vi "Tool Q LEIN High G  Start.vi"(0 "Controller ID":u8=42, 5 "G trigger limit(5 G)":dbl=5.0, 9 "Numb pre samples(250)":u16=250, 11 "error in (no error)":errorcluster) -> (4 "LEIN custom reply Q":T1, 15 "error out":errorcluster)   [LabVIEW 2011]
uses:
  LEINmaster/Defenitions/LEIN custom reply Q.ctl
  LEINmaster/Defenitions/LEIN Reply Holder.ctl
  LEINmaster/Defenitions/LEIN CMD Cluster.ctl
  LEINmaster/Defenitions/LEIN CMD List.ctl
  LEINmaster/Defenitions/LEIN Structure variations.ctl
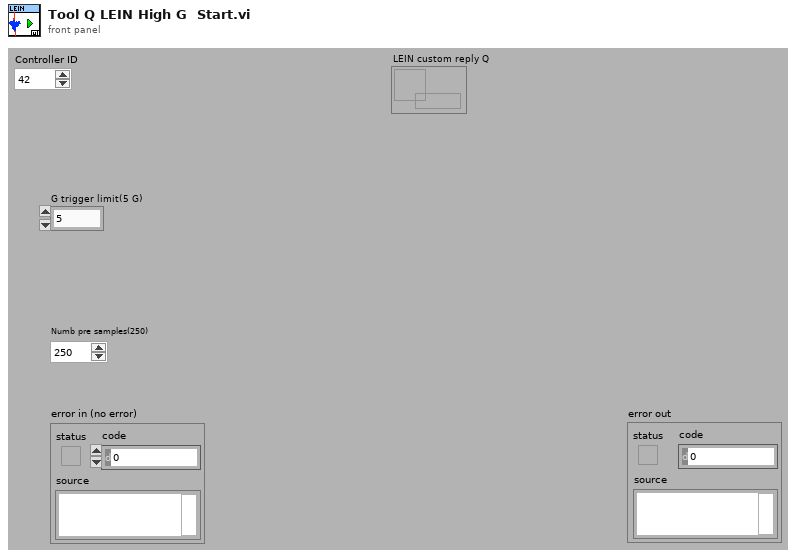
[diagram p1: front panel]
types:
  T1 = typedef "LEIN custom reply Q.ctl" = refnum<queue>
  T2 = typedef "LEIN Structure variations.ctl" = enum16{"LEIN08", "LEIN31", "LEIN63"}
  T3 = enum16{"big-endian, network order", "native, host order", "little-endian"}
  T4 = typedef "LEIN CMD Cluster.ctl" = cluster{"SID":u8, "ANF":bool, "CMD":T5, "DATA":u8[]}
  T5 = typedef "LEIN CMD List.ctl" = enum8{"ACTI", "TASK", "RES0", "STAT", "RES1", "RES2", "RES3", "USER"}
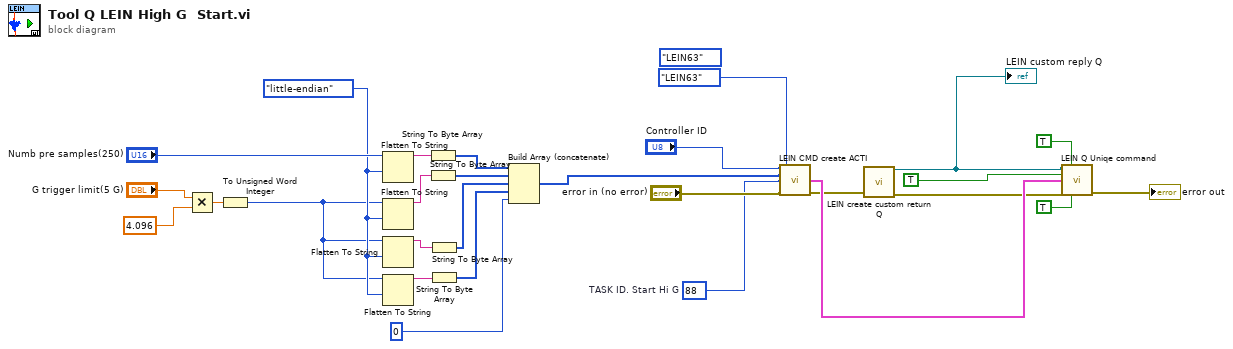
[diagram p0: block diagram]
diagram:
  (unwired) LEIN_Structure_variations."LEIN63" ("LEIN Variation")
  w7 = u8 88  # TASK ID. Start Hi G
  w14 = T3."little-endian" ("byte order (0:big-endian, network order)")
  n1 = Multiply(x="G trigger limit(5 G)", y=4.096 ("x")) -> (x*y=w27:dbl)
  n2 = To Unsigned Word Integer(number=w27) -> (unsigned 16bit integer=w13:u16)
  n3 = Flatten To String(anything="Numb pre samples(250)", byte order (0:big-endian, network order)=w14) -> (data string=w25:string)  [unwired: 2 in, 2 out]
  n4 = Flatten To String(anything=w13, byte order (0:big-endian, network order)=w14) -> (data string=w23:string)  [unwired: 2 in, 2 out]
  n5 = Flatten To String(anything=w13, byte order (0:big-endian, network order)=w14) -> (data string=w17:string)  [unwired: 2 in, 2 out]
  n6 = Flatten To String(anything=w13, byte order (0:big-endian, network order)=w14) -> (data string=w16:string)  [unwired: 2 in, 2 out]
  n7 = String To Byte Array(string=w25) -> (unsigned byte array=w24:u8[])
  n8 = String To Byte Array(string=w23) -> (unsigned byte array=w22:u8[])
  n9 = String To Byte Array(string=w17) -> (unsigned byte array=w18:u8[])
  n10 = String To Byte Array(string=w16) -> (unsigned byte array=w15:u8[])
  n11 = Build Array (concatenate)(w24, w22, w18, w15, u8 0) -> (w8:u8[])
  n12 = call "LEIN CMD create ACTI.vi"("SID"="Controller ID", "LEIN Variation"=LEIN_Structure_variations."LEIN63", "Data"=w8, "ACTI ID"=w7, "error in (no error)"="error in (no error)") -> ("CMD"=w6:T4, "error out"=w5:errorcluster)  [unwired: 9 in]
  n13 = call "LEIN create custom return Q.vi"("error in (no error)"=w5) -> ("LEIN custom reply Q"=w3:T1, "error out"=w4:errorcluster)  [unwired: 13 in]
  "LEIN custom reply Q" <- w3
  n14 = call "LEIN Q Uniqe command.vi"("LEIN custom reply Q"=w3, "Retry on err (F)"=TRUE, "Custom Q(F)"=TRUE, "CMD"=w6, "error in"=w4, "priority(F)"=TRUE) -> ("error out"=→"error out":errorcluster)  [unwired: 9 in]
